vi "ACT_setpoint_tracking.vi"(0 "MD420.lvclass in":refnum<class "MD420.lvclass">, 1 "Target Grad":dbl, 2 "TVal reached":bool, 3 "ACT lower limit":dbl, 4 "ACT limit Setpoint":dbl, 5 "ACT upper limit":dbl, 6 "Rels +0.6 K/min":bool, 7 "error in":errorcluster, 8 "Matching":bool, 10 "-0.9 K/min":bool, 11 "Target Value":dbl) -> (20 "MD420.lvclass out":refnum<class "MD420.lvclass">, 23 "ACT Eff Grad":dbl, 24 "ACT Eff SP":dbl, 27 "error out":errorcluster)   [LabVIEW 2022 SP3, in "MD420.lvclass"]
uses:
  MD420.lvclass
  MD420.lvclass/MD420.ctl
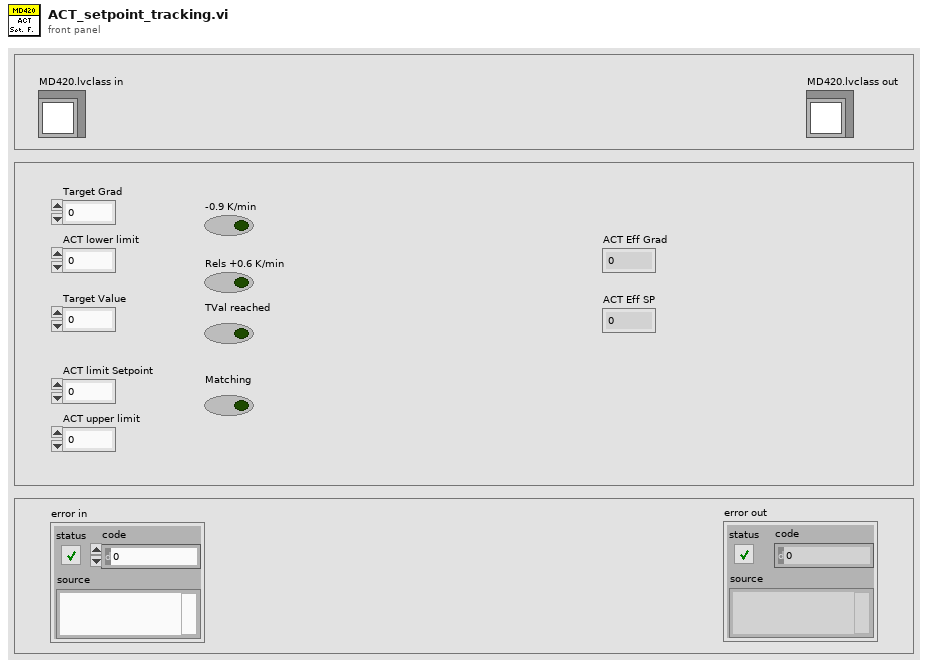
[diagram p1: front panel]
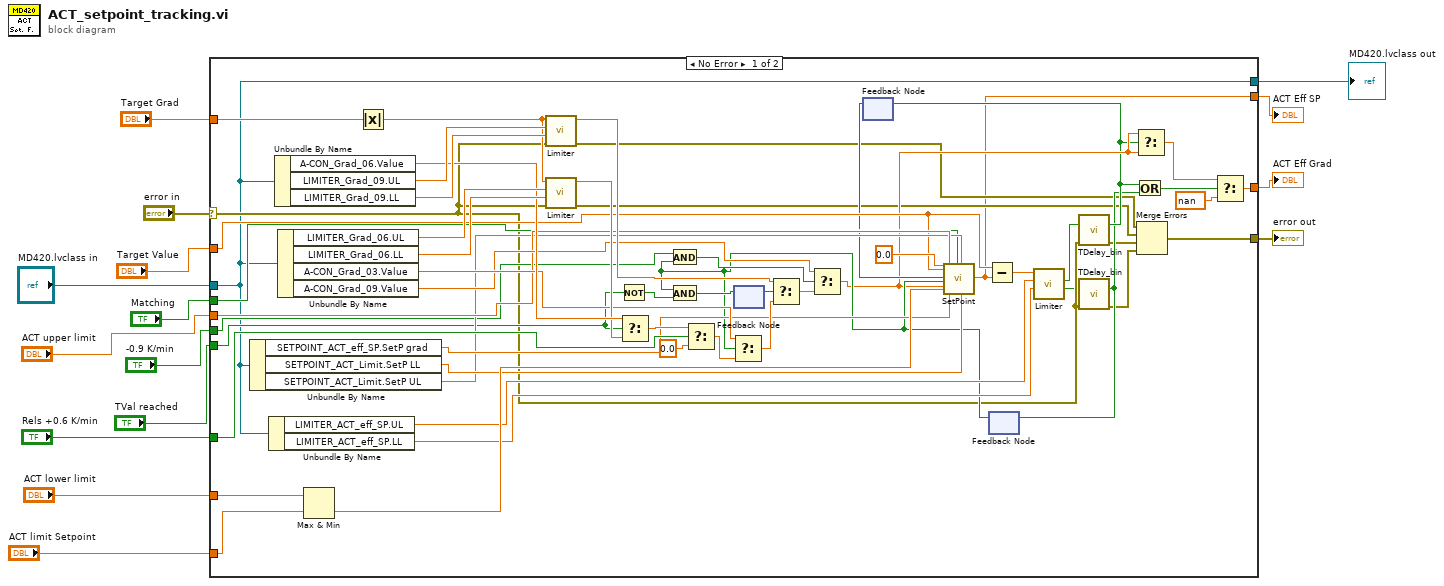
[diagram p0: block diagram]
diagram:
  n1 = case shown="No Error" "error in" {
    selector: "error in" -> [w24 w72]
    tunnel: [w25 w72] -> w14
    tunnel: "MD420.lvclass in" -> [w19 w71]
    tunnel: "Target Grad" -> [w70 _]
    tunnel: "TVal reached" -> [w40 _]
    tunnel: "Rels +0.6 K/min" -> [w62 _]
    tunnel: "ACT upper limit" -> [w49 _]
    tunnel: "ACT lower limit" -> [w53 _]
    tunnel: "ACT limit Setpoint" -> [w52 _]
    tunnel: "Target Value" -> [w45 _]
    tunnel: "Matching" -> [w44 _]
    tunnel: "-0.9 K/min" -> [w38 _]
    tunnel: [w26 _] -> w3
    tunnel: [w19 w71] -> w2
    tunnel: [w18 _] -> w1
    frame No Error {
      n2 = Unbundle By Name(w19) -> ("SETPOINT_ACT_eff_SP.SetP grad"=w48:dbl, "SETPOINT_ACT_Limit.SetP LL"=w47:dbl, "SETPOINT_ACT_Limit.SetP UL"=w46:dbl)
      n3 = Unbundle By Name(w19) -> ("LIMITER_ACT_eff_SP.UL"=w43:dbl, "LIMITER_ACT_eff_SP.LL"=w42:dbl)
      n4 = Unbundle By Name(w19) -> ("A-CON_Grad_06.Value"=w64:dbl, "LIMITER_Grad_09.UL"=w69:dbl, "LIMITER_Grad_09.LL"=w68:dbl)
      n5 = Unbundle By Name(w19) -> ("LIMITER_Grad_06.UL"=w66:dbl, "LIMITER_Grad_06.LL"=w65:dbl, "A-CON_Grad_03.Value"=w59:dbl, "A-CON_Grad_09.Value"=w55:dbl)
      n6 = Max & Min(x=w53, y=w52) -> (min(x,y)=w50:dbl)  [unwired: 1 out]
      n7 = Absolute Value(x=w70) -> (abs(x)=w67:dbl)
      n8 = call "Limiter.vi"("error in"=w24, "LIMITER_PG_lift-up.LL"=w68, "LIMITER_PG_lift-up.UL in"=w69, "input"=w67) -> ("error IO"=w23:errorcluster, "LIMITER_PG_lift-up.UL out"=w56:dbl)  [unwired: 4 in, 2 out]
      n9 = call "Limiter.vi"("error in"=w24, "LIMITER_PG_lift-up.LL"=w65, "LIMITER_PG_lift-up.UL in"=w66, "input"=w67) -> ("error IO"=w22:errorcluster, "LIMITER_PG_lift-up.UL out"=w63:dbl)  [unwired: 4 in, 2 out]
      n10 = Not(x=w40) -> (.not. x?=w39:bool)
      n11 = Select(t=w64, s=w40, f=w63) -> (s? t:f=w61:dbl)
      n12 = Select(t=w61, s=w62, f=0.0) -> (s? t:f=w58:dbl)
      n13 = feedback #1() -> (w36:bool)  [unwired: 1 in]
      n14 = feedback #2() -> (w34:bool)  [unwired: 1 in]
      n15 = feedback #3() -> (w33:bool)  [unwired: 1 in]
      n16 = And(x=w38, y=w33) -> (x .and. y?=w35:bool)
      n17 = And(x=w33, y=w39) -> (x .and. y?=w37:bool)
      n18 = Select(t=w59, s=w33, f=w58) -> (s? t:f=w57:dbl)
      n19 = feedback-in #1(w37) -> ()
      n20 = Select(t=w56, s=w36, f=w57) -> (s? t:f=w54:dbl)
      n21 = Select(t=w55, s=w35, f=w54) -> (s? t:f=w32:dbl)
      n22 = call "SetPoint.vi"("Input"=0.0, "IAd(AI2)"=w45, "I+(BI2)"=w34, "I-(BI1)"=w33, "Igrd(AI1)"=w32, "ILL(AI3)"=w50, "ULL(AI4)"=w49, "SetP Grad"=w48, "IC(BI3)"=w44, "SetP UL"=w46, "SetP LL"=w47) -> ("Output (AO1)"=w18:dbl)  [unwired: 15 in, 1 out]
      n23 = Subtract(x=w45, y=w18) -> (x-y=w41:dbl)
      n24 = call "Limiter.vi"("LIMITER_PG_lift-up.LL"=w42, "LIMITER_PG_lift-up.UL in"=w43, "input"=w41) -> ("low reached"=w16:bool, "upper reached"=w17:bool)  [unwired: 5 in, 2 out]
      n25 = call "TDelay_bin.vi"("Boolean"=w17, "error in"=w24) -> ("output"=w31:bool, "error out"=w21:errorcluster)  [unwired: 12 in]
      n26 = feedback-in #2(w31) -> ()
      n27 = call "TDelay_bin.vi"("Boolean"=w16, "error in"=w24) -> ("output"=w30:bool, "error out"=w20:errorcluster)  [unwired: 12 in]
      n28 = feedback-in #3(w30) -> ()
      n29 = Or(x=w31, y=w30) -> (x .or. y?=w29:bool)
      n30 = Select(t=w32, s=w31, f=w32) -> (s? t:f=w28:dbl)
      n31 = Merge Errors(w23, w22, w21, w20) -> (w25:errorcluster)
      n32 = Select(t=w28, s=w29, f=nan) -> (s? t:f=w26:dbl)
    }
    frame Error {
    }
  }
  "error out" <- w14
  "ACT Eff Grad" <- w3
  "MD420.lvclass out" <- w2
  "ACT Eff SP" <- w1
